vi "while loop concept.vi"() -> ()   [LabVIEW 2018]
panel:
  out "Loop Count 2":i32
  in  "stop 2":bool
  in  "stop":bool
  out "Loop Count":i32
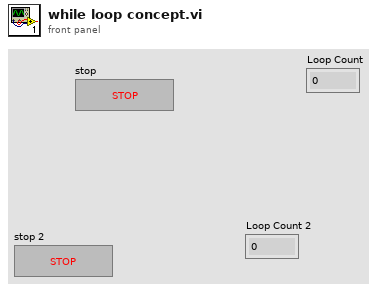
[diagram p1: front panel]
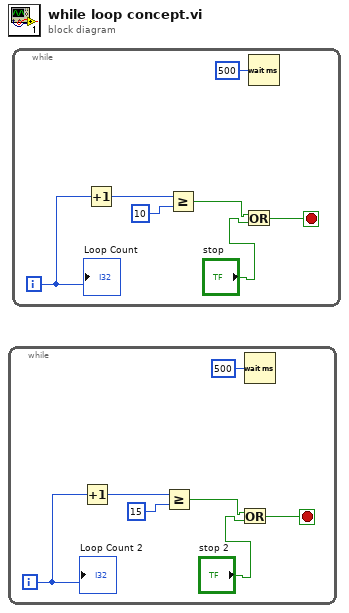
[diagram p0: block diagram]
diagram:
  n1 = while {
    i -> [w2]
    stop <- w3 stop-if-true
    n2 = Increment(x=w2) -> (x+1=w1:i32)
    n3 = Greater Or Equal?(x=w1, y=15) -> (x >= y?=w5:bool)
    n4 = Or(x=w5, y="stop 2") -> (x .or. y?=w3:bool)
    n5 = Wait (ms)(milliseconds to wait=u32 500) -> ()  [unwired: 1 out]
    "Loop Count 2" <- w2
  }
  n6 = while {
    i -> [w9]
    stop <- w10 stop-if-true
    n7 = Increment(x=w9) -> (x+1=w8:i32)
    n8 = Greater Or Equal?(x=w8, y=10) -> (x >= y?=w12:bool)
    n9 = Or(x=w12, y="stop") -> (x .or. y?=w10:bool)
    n10 = Wait (ms)(milliseconds to wait=u32 500) -> ()  [unwired: 1 out]
    "Loop Count" <- w9
  }
